vi "Process.vi"(8 "error in":errorcluster, 11 "SMO":refnum<class "SMO.lvclass">) -> (0 "error out":errorcluster, 3 "SMO out":refnum<class "SMO.lvclass">)   [LabVIEW 2021, in "smo.lvlib" / "SMO.lvclass"]
uses:
  SMO.lvclass
  Typedefs/Parent Call--Enum.ctl
  Typedefs/SMOState --Enum.ctl
  SMO.lvclass/SMO.ctl
  Support/Attribute.ErrorHandling/Attribute.ErrorHandling.lvclass/Attribute.ErrorHandling.ctl
  Support/Attribute.Owner/Packet -- Cluster.ctl
  Support/Attribute/Attribute.lvclass
  Support/Attribute/Attribute.lvclass/Attribute.ctl
  Typedefs/Search Key.ctl
  Private/ReftoDVR--SMO.vi
  Private/GetVariant(Attr).vi
  Support/Attribute.ErrorHandling/Read UnhandledShutdown.vi
  <vilib>/Utility/MD5Checksum.llb/MD5Checksum string.vi
  Support/Attribute.ErrorHandling/Attribute.ErrorHandling.lvclass
  Support/Attribute.Owner/Attribute.Owner.lvclass
panel:
  in  "Test Error":bool
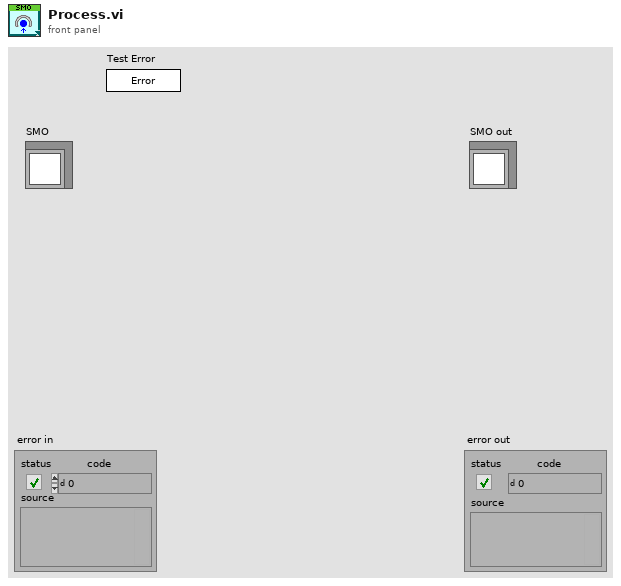
[diagram p1: front panel]
types:
  T1 = typedef "smo.lvlib/SMO.lvclass/SMOState --Enum.ctl" = enum16{"unknown", "Created", "Started", "Stopped"}
  T2 = typedef "smo.lvlib/SMO.lvclass/Parent Call--Enum.ctl" = enum16{"Allows parent to run", "Does not request parent to run"}
  T3 = typedef "smo.lvlib/Attribute.Owner.lvclass/Packet -- Cluster.ctl" = cluster{"Message":string, "Payload":variant, "Source GUID":string}
  T4 = typedef "smo.lvlib/SMO.lvclass/Search Key.ctl" = enum16{"Name", "GUID", "Qualified Name", "Subsystem Path", "Configuration Path"}
  T5 = typedef "smo.lvlib/SMO.lvclass/ProcessRegistrationRefnum.ctl" = refnum<event-registration>
  T6 = cluster{"[Dependencies]":refnum<class "SMO.lvclass">[], "State [Dependencies]":refnum<user-event>[], "Error [Dependencies]":refnum<user-event>[], "Message [Dependencies]":refnum<user-event>[], "Shutdown on Unhandled Error":bool}
  T7 = typedef "SMO.lvclass/SMOState --Enum.ctl" = enum16{"unknown", "Created", "Started", "Stopped"}
  T8 = typedef "smo.lvlib/def.SMO.lvclass/Scope -- Enum.ctl" = enum16{"Public", "Protected", "Private"}
  T9 = typedef "smo.lvlib/SMO.lvclass/SMO Dependency Event--Enum.ctl" = enum16{"Added", "Removed", "Started", "Stopped"}
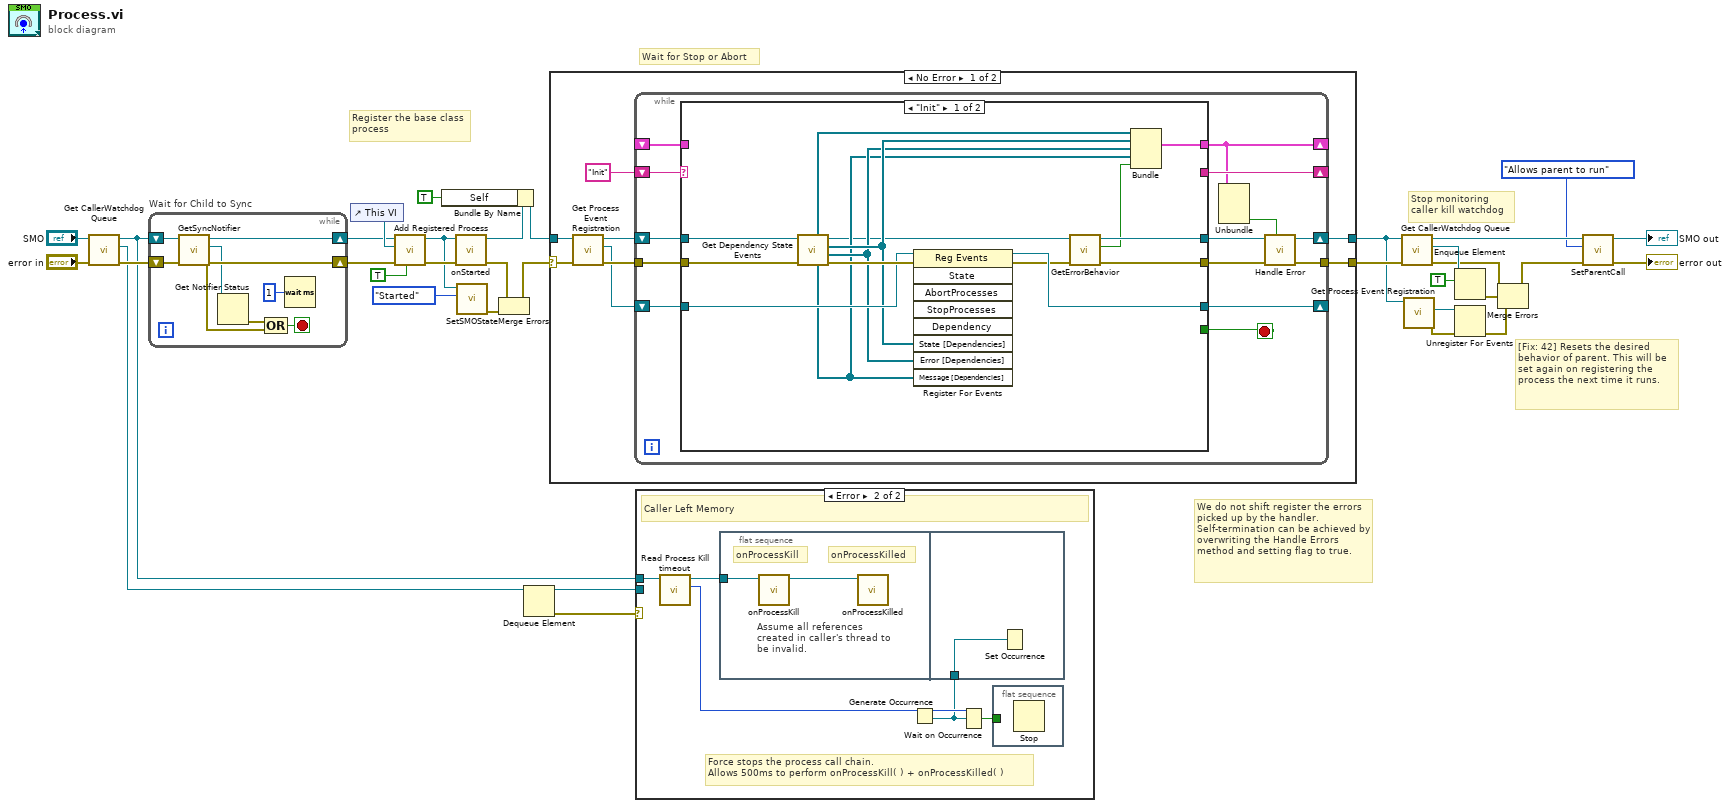
[diagram p0: block diagram]
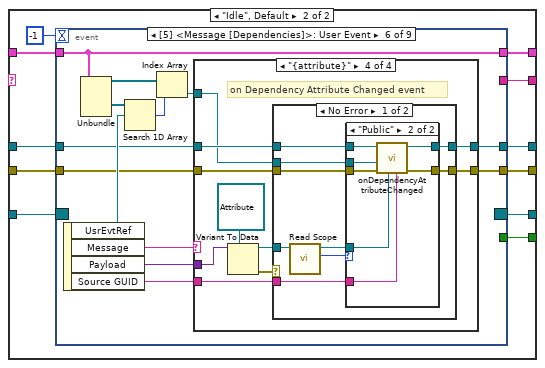
[diagram p3: hidden frame]
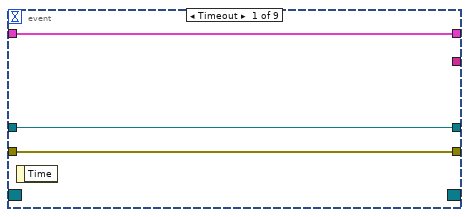
[diagram p4: hidden frame]
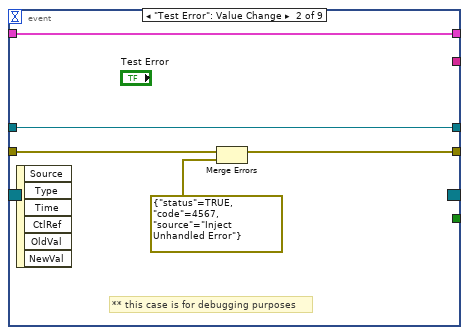
[diagram p5: hidden frame]
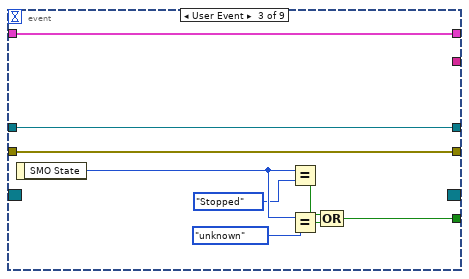
[diagram p6: hidden frame]
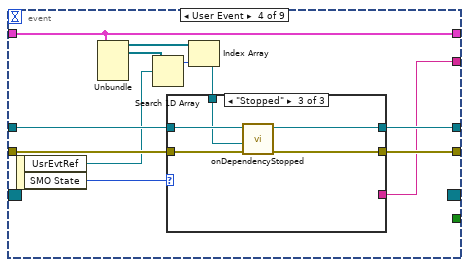
[diagram p7: hidden frame]
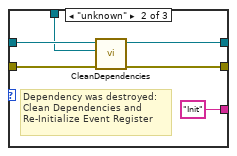
[diagram p9: hidden frame]
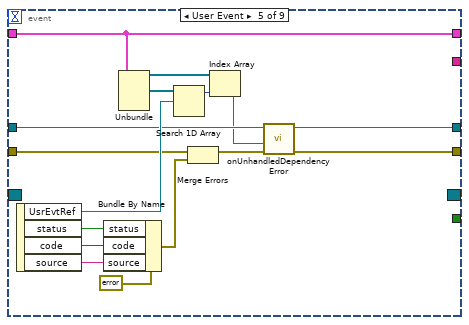
[diagram p10: hidden frame]
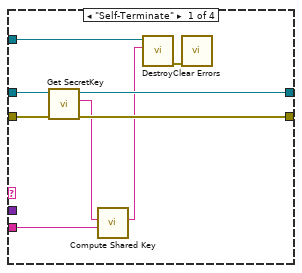
[diagram p11: hidden frame]
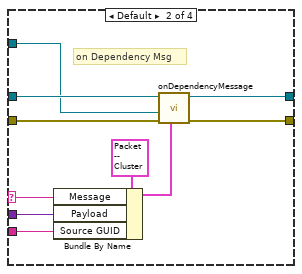
[diagram p12: hidden frame]
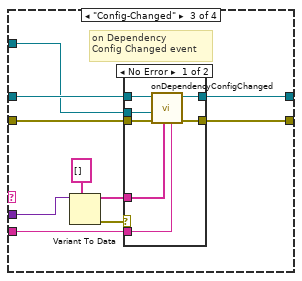
[diagram p13: hidden frame]
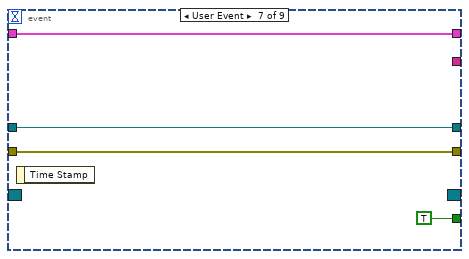
[diagram p17: hidden frame]
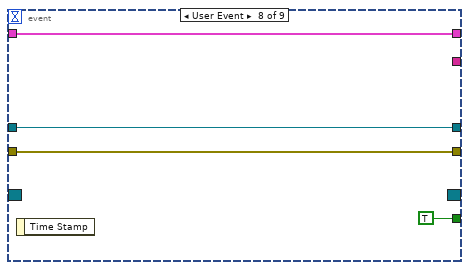
[diagram p18: hidden frame]
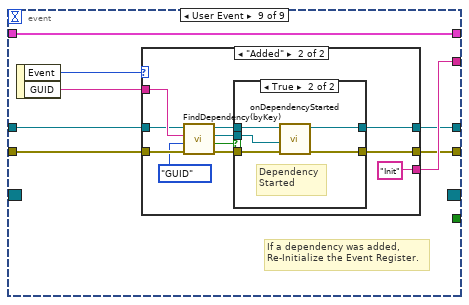
[diagram p19: hidden frame]
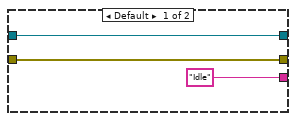
[diagram p20: hidden frame]
diagram:
  # "We do not shift register the errors picked up by the handler. Self-termination can be achieved by overwriting the Handle Errors method and setting flag to true."
  # "[Fix: 42] Resets the desired behavior of parent. This will be set again on registering the process the next time it runs."
  # "Stop monitoring\ncaller kill watchdog"
  # "Wait for Stop or Abort"
  # "Register the base class\nprocess"
  n1 = call "Get CallerWatchdog Queue.vi"("error in (no error)"="error in", "SMO in"="SMO") -> ("error out"=w22:errorcluster, "Caller Watchdog"=w21:refnum<queue>, "SMO out"=w20:refnum<class "SMO.lvclass">)  [unwired: 7 in]
  n2 = while "Wait for Child to Sync" {
    shift-right: [w41] -> w14
    shift-left: w20 -> [w42]
    shift-right: [w38] -> w13
    shift-left: w22 -> [w40]
    stop <- w39 stop-if-true
    n3 = call "GetSyncNotifier.vi"("error in (no error)"=w40, "SMO in"=w42) -> ("error out"=w38:errorcluster, "Sync Notifier"=w36:refnum<notifier>, "SMO out"=w41:refnum<class "SMO.lvclass">)  [unwired: 7 in]
    n4 = Get Notifier Status(notifier=w36) -> (error out=w35:errorcluster)  [unwired: 1 in, 4 out]
    n5 = Compound Arithmetic op=OR(w35, w38) -> (w39:bool)
    n6 = Wait (ms)(milliseconds to wait=u32 1) -> ()  [unwired: 1 out]
  }
  n7 = control-ref of="This VI"() -> (w34:refnum<vi>)
  n8 = call "Add Registered Process.vi"("Process Runs (T)"=TRUE, "error in (no error)"=w13, "Process VI (Static VI Ref)"=w34, "SMO"=w14) -> ("error out"=w32:errorcluster, "SMO out"=w11:refnum<class "SMO.lvclass">)  [unwired: 6 in]
  n9 = call-dynamic "onStarted.vi"("error in (no error)"=w32, "SMO"=w11) -> ("error out"=w9:errorcluster, "SMO out"=w3:refnum<class "SMO.lvclass">)  [unwired: 8 in]
  n10 = Bundle By Name(cluster=w3, "Self"=TRUE ("Reserved.Self")) -> (w2:refnum<class "SMO.lvclass">)
  n11 = call "SetSMOState.vi"("SMO State"=SMOState_--Enum."Started" ("event data"), "SMO in"=w11) -> ("error out"=w10:errorcluster)  [unwired: 8 in, 1 out]
  n12 = Merge Errors(w9, w10) -> (w8:errorcluster)
  n13 = Dequeue Element(queue=w21) -> (queue out=w27:refnum<queue>, error out=w28:errorcluster)  [unwired: 2 in, 2 out]
  n14 = case shown="No Error" w8 {
    selector: w8 -> [w46 w268]
    tunnel: [w50 w268] -> w31
    tunnel: w2 -> [w48 w267]
    tunnel: [w49 w267] -> w7
    frame No Error {
      n15 = call "Get Process Event Registration.vi"("error in (no error)"=w46, "SMO in"=w48) -> ("error out"=w45:errorcluster, "Event Registration Refnum"=w44:T5, "SMO out"=w47:refnum<class "SMO.lvclass">)  [unwired: 7 in]
      n16 = while {
        tunnel: [w55] -> w50
        tunnel: w45 -> [w63]
        shift-right: [w59] -> _
        shift-left: "Init" -> [w58]
        shift-right: [w52] -> _
        shift-left: _ -> [w57]
        shift-right: [w62] -> _
        shift-left: w44 -> [w64]
        shift-right: [w54] -> w49
        shift-left: w47 -> [w61]
        stop <- w60 stop-if-true
        n17 = case shown="\"Init\"" w58 {
          tunnel: [w68 w90] -> w56
          tunnel: w64 -> [w77 w89]
          tunnel: w63 -> [w75 w88]
          tunnel: [w76 w87] -> w62
          tunnel: w61 -> [w78 w86]
          tunnel: [w66 w85] -> w53
          tunnel: [_ w83] -> w60
          tunnel: [_ w82] -> w59
          tunnel: [w71 w80] -> w52
          tunnel: w57 -> [_ w81]
          frame "Init" {
            n18 = call "Get Dependency State Events.vi"("error in (no error)"=w75, "SMO in"=w78) -> ("error out"=w79:errorcluster, "Error [Dependencies]"=w72:refnum<user-event>[], "State [Dependencies]"=w73:refnum<user-event>[], "SMO out"=w67:refnum<class "SMO.lvclass">, "Message [Dependencies]"=w70:refnum<user-event>[], "[Dependencies]"=w74:refnum<class "SMO.lvclass">[])  [unwired: 4 in]
            n19 = register-events(reference=w77, error in=w79, w73, w72, w70) -> (reference out=w76:T5, error out=w69:errorcluster)  [unwired: 4 in]
            n20 = call "GetErrorBehavior.vi"("error in (no error)"=w69, "SMO in"=w67) -> ("error out"=w68:errorcluster, "Shutdown on Unhandled Error"=w65:bool, "SMO out"=w66:refnum<class "SMO.lvclass">)  [unwired: 7 in]
            n21 = Bundle("[Dependencies]"=w74, "State [Dependencies]"=w73, "Error [Dependencies]"=w72, "Message [Dependencies]"=w70, "Shutdown on Unhandled Error"=w65) -> (w71:T6)  [unwired: 1 in]
          }
          frame "Idle", Default {
            n22 = event shown="[5] <Message [Dependencies]>: User Event" {
              selector: w89 -> [_ _ _ _ _ _ _ _ _]
              dyn-events: [_ _ _ _ _ _ _ _ _] -> w87
              timeout: -1 -> [_ _ _ _ _ _ _ _ _]
              tunnel: w88 -> [w92 w96 w107 w115 w137 w154 w232 w236 w239]
              tunnel: [w92 w94 w107 w116 w134 w153 w232 w236 w240] -> w90
              tunnel: w86 -> [w93 w95 w103 w118 w139 w156 w233 w237 w242]
              tunnel: [w93 w95 w103 w117 w133 w155 w233 w237 w241] -> w85
              tunnel: [_ _ w100 _ _ _ TRUE TRUE _] -> w83
              tunnel: [_ _ _ w114 _ _ _ _ w243] -> w82
              tunnel: w81 -> [w91 w98 w99 w111 w144 w161 w230 w234 w245]
              tunnel: [w91 w98 w99 w111 w144 w161 w230 w234 w245] -> w80
              event Timeout {
                n23 = event-data() -> ()  [unwired: 1 in, 1 out]
              }
              event "Test Error": Value Change {
                # "** this case is for debugging purposes"
                n24 = event-data() -> ()  [unwired: 1 in, 6 out]
                n25 = Merge Errors(w96, errorcluster {"status"=TRUE, "code"=4567, "source"="Inject Unhandled Error"} ("error in")) -> (w94:errorcluster)
              }
              event User Event {
                n26 = event-data() -> ("SMO State"=w102:T1)  [unwired: 1 in]
                n27 = Equal?(x=w102, y=SMOState_--Enum."Stopped") -> (x = y?=w105:bool)
                n28 = Equal?(x=w102, y=SMOState_--Enum."unknown") -> (x = y?=w106:bool)
                n29 = Compound Arithmetic op=OR(w105, w106) -> (w100:bool)
              }
              event User Event {
                n30 = event-data() -> ("UsrEvtRef"=w109:refnum<user-event>, "SMO State"=w119:T7)  [unwired: 1 in]
                n31 = Unbundle(w111) -> ("[Dependencies]"=w112:refnum<class "SMO.lvclass">[], "State [Dependencies]"=w110:refnum<user-event>[])  [unwired: 3 out]
                n32 = Search 1D Array(1D array=w110, element=w109) -> (index of element=w113:i32)  [unwired: 1 in]
                n33 = Index Array(array=w112, index=w113) -> (element=w108:refnum<class "SMO.lvclass">)
                n34 = case shown="\"Stopped\"" w119 {
                  tunnel: w118 -> [w121 w127 w132]
                  tunnel: [w121 w126 w130] -> w117
                  tunnel: [w120 w124 w128] -> w116
                  tunnel: w115 -> [w120 w125 w129]
                  tunnel: [_ "Init" _] -> w114
                  tunnel: w108 -> [_ w122 w131]
                  frame Default {
                  }
                  frame "unknown" {
                    # "Dependency was destroyed:\nClean Dependencies and\nRe-Initialize Event Register"
                    n35 = call "CleanDependencies.vi"("error in (no error)"=w125, "Dependency"=w122, "SMO in"=w127) -> ("error out"=w124:errorcluster, "SMO out"=w126:refnum<class "SMO.lvclass">)  [unwired: 6 in, 1 out]
                  }
                  frame "Stopped" {
                    n36 = call-dynamic "onDependencyStopped.vi"("error in"=w129, "Dependency"=w131, "SMO in"=w132) -> ("error out"=w128:errorcluster, "SMO out"=w130:refnum<class "SMO.lvclass">)  [unwired: 7 in]
                  }
                }
              }
              event User Event {
                n37 = event-data() -> ("UsrEvtRef"=w142:refnum<user-event>, "status"=w145:bool, "code"=w146:i32, "source"=w147:string)  [unwired: 1 in]
                n38 = Bundle By Name(cluster=errorcluster {"status"=FALSE, "code"=0, "source"=""} ("error constant"), "status"=w145, "code"=w146, "source"=w147) -> (w135:errorcluster)
                n39 = Unbundle(w144) -> ("[Dependencies]"=w141:refnum<class "SMO.lvclass">[], "Error [Dependencies]"=w143:refnum<user-event>[])  [unwired: 3 out]
                n40 = Search 1D Array(1D array=w143, element=w142) -> (index of element=w140:i32)  [unwired: 1 in]
                n41 = Merge Errors(w137, w135) -> (w136:errorcluster)
                n42 = Index Array(array=w141, index=w140) -> (element=w138:refnum<class "SMO.lvclass">)
                n43 = call-dynamic "onUnhandledDependencyError.vi"("Unhandled Dependency Error"=w136, "Dependency"=w138, "SMO in"=w139) -> ("Unhandled error"=w134:errorcluster, "SMO out"=w133:refnum<class "SMO.lvclass">)  [unwired: 7 in]
              }
              event User Event {
                n44 = event-data() -> ("UsrEvtRef"=w160:refnum<user-event>, "Message"=w157:string, "Payload"=w150:variant, "Source GUID"=w151:string)  [unwired: 1 in]
                n45 = Unbundle(w161) -> ("[Dependencies]"=w159:refnum<class "SMO.lvclass">[], "Message [Dependencies]"=w158:refnum<user-event>[])  [unwired: 3 out]
                n46 = Search 1D Array(1D array=w158, element=w160) -> (index of element=w149:i32)  [unwired: 1 in]
                n47 = Index Array(array=w159, index=w149) -> (element=w152:refnum<class "SMO.lvclass">)
                n48 = case shown="\"{attribute}\"" w157 {
                  selector: w157 -> [_ w174 _ _]
                  tunnel: w156 -> [w170 w180 w190 w209]
                  tunnel: [w169 w171 w189 w208] -> w155
                  tunnel: w154 -> [w168 w179 w188 w207]
                  tunnel: [w167 w178 w186 w205] -> w153
                  tunnel: w152 -> [w165 w177 w187 w206]
                  tunnel: w151 -> [w166 w172 w185 w204]
                  tunnel: w150 -> [_ w173 w184 w203]
                  frame "Self-Terminate" {
                    n49 = call "Get SecretKey.vi"("error in (no error)"=w168, "SMO"=w170) -> ("error out"=w167:errorcluster, "SecretKey"=w162:string, "SMO out"=w169:refnum<class "SMO.lvclass">)  [unwired: 7 in]
                    n50 = call "Compute Shared Key.vi"("GUID"=w166, "SecretKey"=w162) -> ("Shared Key"=w164:string)  [unwired: 9 in]
                    n51 = call "Destroy.vi"("Shared Key"=w164, "SMO"=w165) -> ("error out"=w163:errorcluster)  [unwired: 9 in]
                    n52 = call <vilib>:"Clear Errors.vi"("error in (no error)"=w163) -> ()  [unwired: 5 in, 2 out]
                  }
                  frame Default {
                    # "on Dependency Msg"
                    n53 = Bundle By Name(cluster=T3 {"Message"="", "Payload"=variant, "Source GUID"=""} ("Packet"), "Message"=w174, "Payload"=w173, "Source GUID"=w172) -> (w176:T3)
                    n54 = call-dynamic "onDependencyMessage.vi"("Packet"=w176, "error in"=w179, "Dependency"=w177, "SMO in"=w180) -> ("error out"=w178:errorcluster, "SMO out"=w171:refnum<class "SMO.lvclass">)  [unwired: 6 in]
                  }
                  frame "Config-Changed" {
                    # "on Dependency\nConfig Changed event"
                    n55 = Variant To Data(type=string[] [] ("keys changed"), Variant=w184) -> (data=w182:string[], error out=w181:errorcluster)  [unwired: 1 in]
                    n56 = case shown="No Error" w181 {
                      tunnel: w190 -> [w197 w199]
                      tunnel: [w196 w199] -> w189
                      tunnel: w188 -> [w195 w198]
                      tunnel: w187 -> [w194 _]
                      tunnel: [w193 w198] -> w186
                      tunnel: w185 -> [w192 _]
                      tunnel: w182 -> [w191 _]
                      frame No Error {
                        n57 = call-dynamic "onDependencyConfigChanged.vi"("Source GUID"=w192, "keys changed"=w191, "error in"=w195, "Dependency"=w194, "SMO in"=w197) -> ("error out"=w193:errorcluster, "SMO out"=w196:refnum<class "SMO.lvclass">)  [unwired: 5 in]
                      }
                      frame Error {
                      }
                    }
                  }
                  frame "{attribute}" {
                    # "on Dependency Attribute Changed event"
                    n58 = Variant To Data(type=refnum<class "Attribute.lvclass"> refnum ("Attribute"), Variant=w203) -> (data=w202:refnum<class "Attribute.lvclass">, error out=w201:errorcluster)  [unwired: 1 in]
                    n59 = case shown="No Error" w201 {
                      tunnel: w209 -> [w218 w229]
                      tunnel: [w217 w229] -> w208
                      tunnel: w207 -> [w215 w228]
                      tunnel: w206 -> [w214 _]
                      tunnel: [w216 w228] -> w205
                      tunnel: w204 -> [w213 _]
                      tunnel: w202 -> [w212 _]
                      frame No Error {
                        n60 = call "Read Scope.vi"("Attribute in"=w212) -> ("Scope"=w210:T8, "Attribute out"=w211:refnum<class "Attribute.lvclass">)  [unwired: 9 in]
                        n61 = case shown="\"Public\"" w210 {
                          tunnel: w218 -> [w220 w227]
                          tunnel: [w220 w226] -> w217
                          tunnel: [w219 w225] -> w216
                          tunnel: w215 -> [w219 w224]
                          tunnel: w214 -> [_ w223]
                          tunnel: w213 -> [_ w222]
                          tunnel: w211 -> [_ w221]
                          frame Default {
                          }
                          frame "Public" {
                            n62 = call-dynamic "onDependencyAttributeChanged.vi"("Source GUID"=w222, "Attribute"=w221, "error in"=w224, "Dependency"=w223, "SMO in"=w227) -> ("error out"=w225:errorcluster, "SMO out"=w226:refnum<class "SMO.lvclass">)  [unwired: 5 in]
                          }
                        }
                      }
                      frame Error {
                      }
                    }
                  }
                }
              }
              event User Event {
                n63 = event-data() -> ()  [unwired: 1 in, 1 out]
              }
              event User Event {
                n64 = event-data() -> ()  [unwired: 1 in, 1 out]
              }
              event User Event {
                # "If a dependency was added,\nRe-Initialize the Event Register."
                n65 = event-data() -> ("Event"=w244:T9, "GUID"=w238:string)  [unwired: 1 in]
                n66 = case shown="\"Added\"" w244 {
                  tunnel: ["Idle" "Init"] -> w243
                  tunnel: w242 -> [w247 w257]
                  tunnel: [w247 w251] -> w241
                  tunnel: [w246 w250] -> w240
                  tunnel: w239 -> [w246 w256]
                  tunnel: w238 -> [_ w258]
                  frame Default {
                  }
                  frame "Added" {
                    n67 = call "FindDependency(byKey).vi"("error in (no error)"=w256, "Search Key (Name)"=Search_Key."GUID", "Key"=w258, "SMO in"=w257) -> ("error out"=w253:errorcluster, "Found?"=w254:bool, "Dependency"=w249:refnum<class "SMO.lvclass">, "SMO dup"=w252:refnum<class "SMO.lvclass">)  [unwired: 4 in]
                    n68 = case shown="True" w254 {
                      tunnel: w253 -> [w260 w263]
                      tunnel: w252 -> [w261 w266]
                      tunnel: [w261 w264] -> w251
                      tunnel: [w260 w262] -> w250
                      tunnel: w249 -> [_ w265]
                      frame False {
                      }
                      frame True {
                        # "Dependency\nStarted"
                        n69 = call-dynamic "onDependencyStarted.vi"("error in"=w263, "Dependency"=w265, "SMO in"=w266) -> ("error out"=w262:errorcluster, "SMO out"=w264:refnum<class "SMO.lvclass">)  [unwired: 7 in]
                      }
                    }
                  }
                }
              }
            }
          }
        }
        n70 = Unbundle(w52) -> ("Shutdown on Unhandled Error"=w51:bool)  [unwired: 4 out]
        n71 = call-dynamic "Handle Error.vi"("Stop on Unhandled Error (T)"=w51, "error in"=w56, "SMO"=w53) -> ("handling error"=w55:errorcluster, "SMO out"=w54:refnum<class "SMO.lvclass">)  [unwired: 6 in, 1 out]
      }
    }
    frame Error {
    }
  }
  n72 = case shown="Error" w28 {
    tunnel: w27 -> [_ _]
    tunnel: w20 -> [_ w272]
    frame No Error {
      # "Process Terminated Normally"
    }
    frame Error {
      # "Force stops the process call chain.\nAllows 500ms to perform onProcessKill( ) + onProcessKilled( )"
      # "Caller Left Memory"
      n73 = call "Read Process Kill timeout.vi"("SMO in"=w272) -> ("Process Kill timeout (ms)"=w270:i32, "SMO out"=w271:refnum<class "SMO.lvclass">)  [unwired: 9 in]
      n74 = flat-sequence {
        tunnel: w271 -> [w275]
        tunnel: w269 -> [w276]
        frame #0 {
          # "Assume all references created in caller's thread to be invalid."
          # "onProcessKilled"
          # "onProcessKill"
          n75 = call-dynamic "onProcessKill.vi"("SMO in"=w275) -> ("SMO out"=w274:refnum<class "SMO.lvclass">)  [unwired: 10 in]
          n76 = call-dynamic "onProcessKilled.vi"("SMO in"=w274) -> ()  [unwired: 11 in]
        }
        frame #1 {
          n77 = Set Occurrence(w276) -> ()
        }
      }
      n78 = Generate Occurrence() -> (w269:refnum<k4>)
      n79 = Wait on Occurrence(2:w269, 3:w270) -> (0:w273:bool)  [unwired: 1 in]
      n80 = flat-sequence {
        tunnel: w273 -> [_]
        frame #0 {
          n81 = Stop() -> ()  [unwired: 1 in]
        }
      }
    }
  }
  n82 = call "Get CallerWatchdog Queue.vi"("error in (no error)"=w31, "SMO in"=w7) -> ("error out"=w25:errorcluster, "Caller Watchdog"=w30:refnum<queue>, "SMO out"=w17:refnum<class "SMO.lvclass">)  [unwired: 7 in]
  n83 = call "Get Process Event Registration.vi"("SMO in"=w7) -> ("error out"=w4:errorcluster, "Event Registration Refnum"=w6:T5)  [unwired: 8 in, 1 out]
  n84 = Enqueue Element(queue=w30, element=TRUE) -> (error out=w26:errorcluster)  [unwired: 2 in, 2 out]
  n85 = Unregister For Events(event registration refnum=w6, error in=w4) -> (error out=w5:errorcluster)
  n86 = Merge Errors(w25, w26, w5) -> (w19:errorcluster)
  n87 = call "SetParentCall.vi"("error in (no error)"=w19, "Parent Call"=Parent_Call--Enum."Allows parent to run", "SMO in"=w17) -> ("error out"=→"error out":errorcluster, "SMO out"=→"SMO out":refnum<class "SMO.lvclass">)  [unwired: 7 in]
